vi "Write Colour.vi"(8 "error in (no error)":errorcluster, 10 "Colour":u32(colorbox), 11 "GameEl in":refnum<class "GameEl.lvclass">) -> (0 "error out":errorcluster, 3 "GameEl out":refnum<class "GameEl.lvclass">)   [LabVIEW 2021, in "GameEl.lvclass"]
uses:
  GameEl.lvclass
  GameEl.lvclass/GameEl.ctl
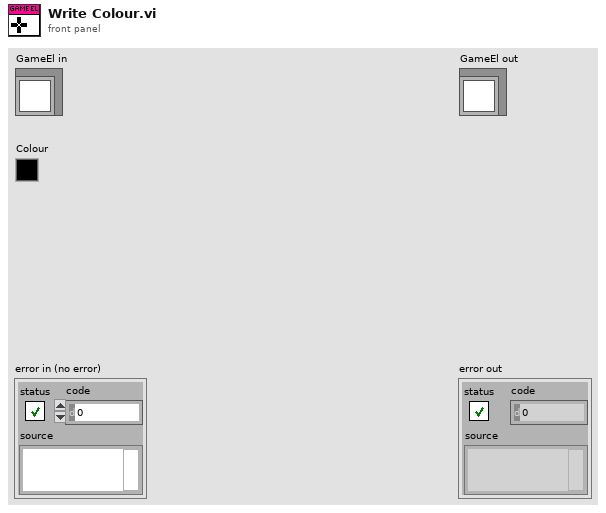
[diagram p1: front panel]
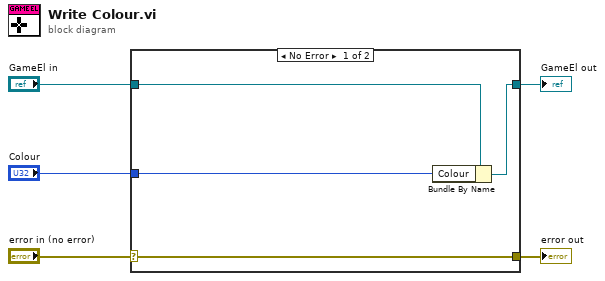
[diagram p0: block diagram]
diagram:
  n1 = case shown="No Error" "error in (no error)" {
    selector: "error in (no error)" -> [w9 w10]
    tunnel: [w9 w10] -> w4
    tunnel: [w7 w11] -> w2
    tunnel: "GameEl in" -> [w8 w11]
    tunnel: "Colour" -> [w6 _]
    frame No Error {
      n2 = Bundle By Name(cluster=w8, "Colour"=w6) -> (w7:refnum<class "GameEl.lvclass">)
    }
    frame Error {
    }
  }
  "error out" <- w4
  "GameEl out" <- w2
